vi "GetComponentStats.vi"(6 "+/-sigmaBounds":dbl=3.0, 11 "Vmag         U             V             W          Cone":dbl[][](array[numeric]) caption="VmagUVWConeData") -> (2 "Stats":dbl[][](array[numeric]))   [LabVIEW 2016]
uses:
  <vilib>/gmath/NI_Gmath.lvlib
  <vilib>/Analysis/NI_AALBase.lvlib
panel:
  # "Mean"
  # "Sigma"
  # "Skew"
  # "Kurt"
  # "MaxBound"
  # "MinBound"
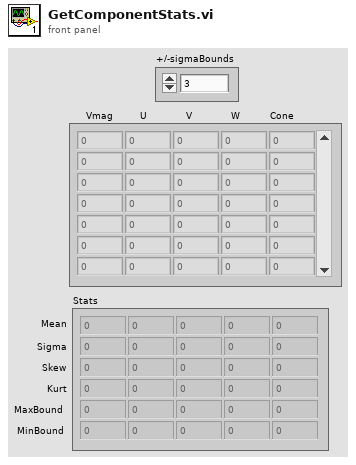
[diagram p1: front panel]
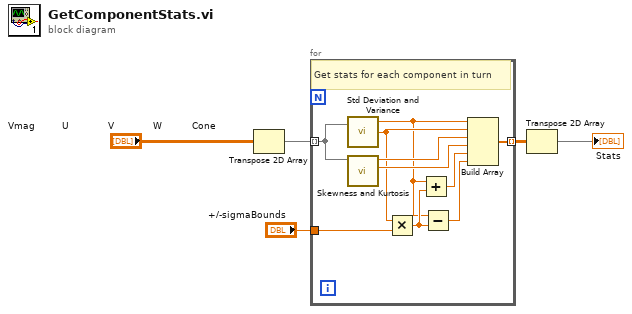
[diagram p0: block diagram]
diagram:
  n1 = Transpose 2D Array(2D array="Vmag         U             V             W          Cone") -> (transposed array=w4:dbl[][])
  n2 = for {
    tunnel: w4 -> [w13] mode=indexing
    tunnel: [w12] -> w3 mode=indexing
    tunnel: "+/-sigmaBounds" -> [w11]
    # "Get stats for each component in turn"
    n3 = call <vilib>:"Std Deviation and Variance.vi"("X"=w13) -> ("mean"=w7:dbl, "standard deviation"=w10:dbl)  [unwired: 1 in, 1 out]
    n4 = call <vilib>:"Skewness and Kurtosis.vi"("X"=w13) -> ("kurtosis"=w14:dbl, "skewness"=w15:dbl)  [unwired: 8 in, 1 out]
    n5 = Multiply(x=w10, y=w11) -> (x*y=w8:dbl)
    n6 = Add(x=w7, y=w8) -> (x+y=w9:dbl)
    n7 = Subtract(x=w7, y=w8) -> (x-y=w6:dbl)
    n8 = Build Array(w7, w10, w15, w14, w9, w6) -> (w12:dbl[])
  }
  n9 = Transpose 2D Array(2D array=w3) -> (transposed array=→"Stats":dbl[][])
